vi "Draw.vi"(8 "error in (no error)":errorcluster, 10 "Picture in":picture, 11 "Triangle in":refnum<class "Triangle.lvclass">) -> (0 "error out":errorcluster, 2 "Picture out":picture, 3 "Triangle out":refnum<class "Triangle.lvclass">)   [LabVIEW 2015, in "Triangle.lvclass"]
uses:
  Triangle.lvclass
  Graphic/Graphic.lvclass/Graphic.ctl
  Line/Line.lvclass
  Polygon/Polygon.lvclass/Polygon.ctl
  Polygon/Polygon.lvclass
  Graphic/Graphic.lvclass
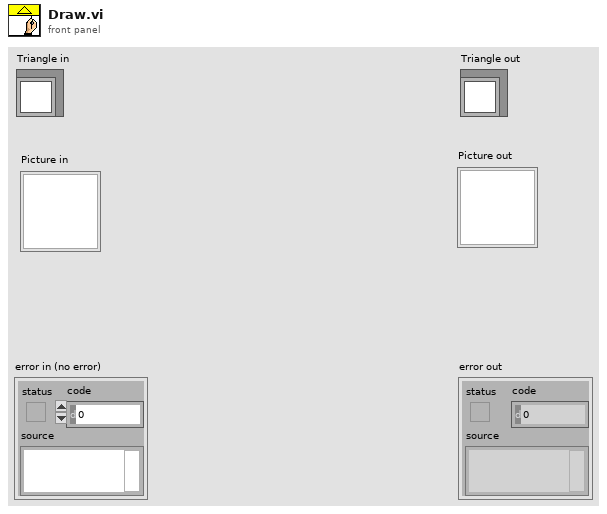
[diagram p1: front panel]
types:
  T1 = typedef "Graphic.lvclass/Style.ctl" = cluster{"Color":u32, "Pen":cluster{"Width":u16, "Style":enum32{"Solid", "Dash", "Dot", "DashDot", "DashDotDot"}}}
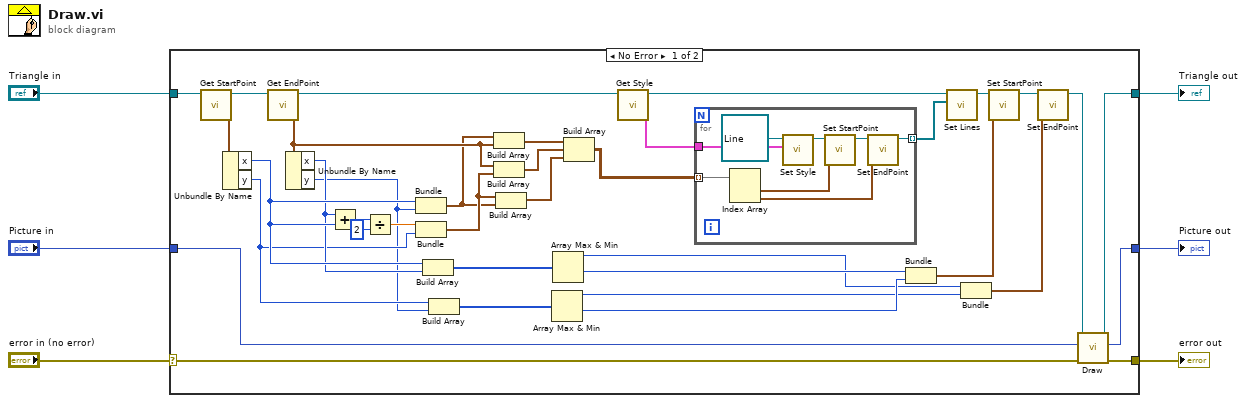
[diagram p0: block diagram]
diagram:
  n1 = case shown="No Error" "error in (no error)" {
    selector: "error in (no error)" -> [w40 w54]
    tunnel: [w43 w54] -> w6
    tunnel: [w42 w52] -> w5
    tunnel: [w41 w53] -> w4
    tunnel: "Picture in" -> [w39 w52]
    tunnel: "Triangle in" -> [w38 w53]
    frame No Error {
      n2 = call "Get StartPoint.vi"("Graphic in"=w38) -> ("StartPoint"=w35:cluster{"x":i16, "y":i16}, "Graphic out"=w37:refnum<class "Triangle.lvclass">)  [unwired: 8 in, 1 out]
      n3 = Unbundle By Name(w35) -> ("x"=w17:i16, "y"=w15:i16)
      n4 = call "Get EndPoint.vi"("Graphic in"=w37) -> ("EndPoint"=w31:cluster{"x":i16, "y":i16}, "Graphic out"=w36:refnum<class "Triangle.lvclass">)  [unwired: 8 in, 1 out]
      n5 = Unbundle By Name(w31) -> ("x"=w16:i16, "y"=w14:i16)
      n6 = Add(x=w16, y=w17) -> (x+y=w34:i16)
      n7 = Divide(x=w34, y=i16 2) -> (x/y=w32:dbl)
      n8 = Bundle("x"=w17, "y"=w14) -> (w29:cluster{"x":i16, "y":i16})  [unwired: 1 in]
      n9 = Bundle(w32, "y"=w15) -> (w30:cluster{dbl, "y":i16})  [unwired: 1 in]
      n10 = Build Array(w17, w16) -> (w23:i16[])
      n11 = Build Array(w15, w14) -> (w22:i16[])
      n12 = Build Array(w29, w31) -> (w28:cluster{"x":i16, "y":i16}[])
      n13 = Build Array(w31, w30) -> (w27:cluster{"x":dbl, "y":i16}[])
      n14 = Build Array(w30, w29) -> (w26:cluster{"x":dbl, "y":i16}[])
      n15 = Array Max & Min(array=w22) -> (max value=w18:i16, min value=w20:i16)  [unwired: 2 out]
      n16 = Array Max & Min(array=w23) -> (max value=w19:i16, min value=w21:i16)  [unwired: 2 out]
      n17 = Build Array(w28, w27, w26) -> (w25:cluster{"x":dbl, "y":i16}[][])
      n18 = call "Get Style.vi"("Graphic in"=w36) -> ("Style"=w7:T1, "Graphic out"=w8:refnum<class "Triangle.lvclass">)  [unwired: 8 in, 1 out]
      n19 = for {
        tunnel: w25 -> [w49] mode=indexing
        tunnel: [w46] -> w24 mode=indexing
        tunnel: w7 -> [w44]
        n20 = Index Array(array=w49) -> (element #1=w48:cluster{"x":dbl, "y":i16}, element #2=w47:cluster{"x":dbl, "y":i16})  [unwired: 2 in]
        n21 = call "Set Style.vi"("Style"=w44, "Graphic in"=refnum<class "Line.lvclass"> refnum ("Line.lvclass")) -> ("Graphic out"=w45:refnum<class "Line.lvclass">)  [unwired: 8 in, 1 out]
        n22 = call "Set StartPoint.vi"("StartPoint"=w48, "Graphic in"=w45) -> ("Graphic out"=w50:refnum<class "Line.lvclass">)  [unwired: 8 in, 1 out]
        n23 = call "Set EndPoint.vi"("EndPoint"=w47, "Graphic in"=w50) -> ("Graphic out"=w46:refnum<class "Line.lvclass">)  [unwired: 8 in, 1 out]
      }
      n24 = Bundle(w21, w20) -> (w10:cluster{i16, i16})  [unwired: 1 in]
      n25 = call "Set Lines.vi"("Lines"=w24, "Polygon in"=w8) -> ("Polygon out"=w13:refnum<class "Triangle.lvclass">)  [unwired: 8 in, 1 out]
      n26 = Bundle(w19, w18) -> (w9:cluster{i16, i16})  [unwired: 1 in]
      n27 = call "Set StartPoint.vi"("StartPoint"=w10, "Graphic in"=w13) -> ("Graphic out"=w12:refnum<class "Triangle.lvclass">)  [unwired: 8 in, 1 out]
      n28 = call "Set EndPoint.vi"("EndPoint"=w9, "Graphic in"=w12) -> ("Graphic out"=w11:refnum<class "Triangle.lvclass">)  [unwired: 8 in, 1 out]
      n29 = call-parent "Draw.vi"("error in (no error)"=w40, "Picture in"=w39, "Polygon in"=w11) -> ("error out"=w43:errorcluster, "Picture out"=w42:picture, "Polygon out"=w41:refnum<class "Triangle.lvclass">)  [unwired: 6 in]
    }
    frame Error {
    }
  }
  "error out" <- w6
  "Triangle out" <- w4
  "Picture out" <- w5
